vi "URAPI_ForStart.vi"(0 "Iterations":string, 3 "URAPI Script":T1={"Script"="", "Whiles"=[], "Ifs"=[], "Supress Err"=TRUE, "Errors"=""}) -> (2 "variable":string, 5 "URAPI Script Out":T1={"Script"="", "Whiles"=[], "Ifs"=[], "Supress Err"=TRUE, "Errors"=""})   [LabVIEW 2012]
doc: "Begins the execution of a for loop. The loop will execute the specified number of \"iterations\".\nNote: requires Loop end VI."
uses:
  <userlib>/BotSpeak/VIs/Direct/URAPI_Control.ctl
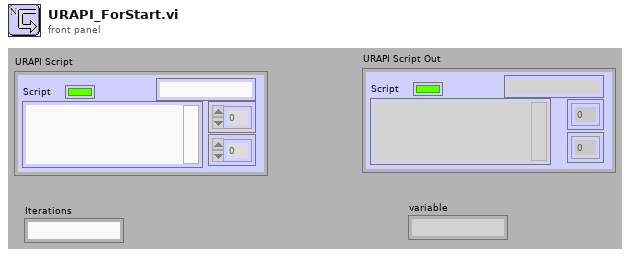
[diagram p1: front panel]
types:
  T1 = typedef "URAPI_Control.ctl" = cluster{"Script":string, "Whiles":u8[], "Ifs":u8[], "Supress Err":bool, "Errors":string}
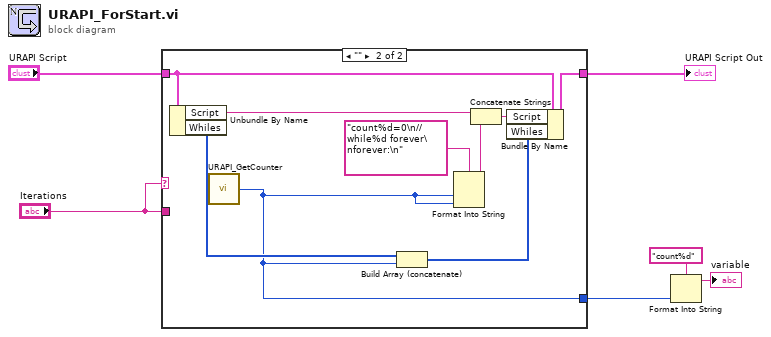
[diagram p0: block diagram]
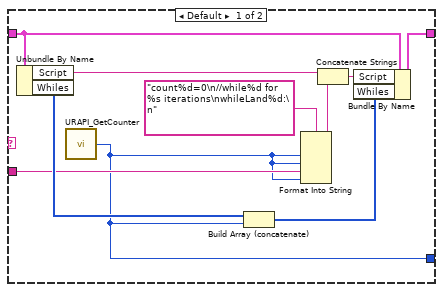
[diagram p2: hidden frame]
diagram:
  n1 = case shown="\"\"" "Iterations" {
    tunnel: "URAPI Script" -> [w16 w25]
    tunnel: [w14 w23] -> w6
    tunnel: "Iterations" -> [w8 _]
    tunnel: [w7 w17] -> w4
    frame Default {
      n2 = Unbundle By Name(w16) -> ("Script"=w11:string, "Whiles"=w10:u8[])
      n3 = call <userlib>:"URAPI_GetCounter.vi"() -> ("Numeric"=w7:u16)  [unwired: 1 in]
      n4 = Build Array (concatenate)(w10, w7) -> (w9:u16[])
      n5 = Format Into String(format string="count%d=0\n//while%d for %s iterations\nwhileLand%d:\n" ("string"), w7, w7, w8, w7) -> (resulting string=w12:string)  [unwired: 2 in, 1 out]
      n6 = Concatenate Strings(w11, w12) -> (w15:string)
      n7 = Bundle By Name(cluster=w16, "Script"=w15, "Whiles"=w9) -> (w14:T1)
    }
    frame "" {
      n8 = Unbundle By Name(w25) -> ("Script"=w20:string, "Whiles"=w19:u8[])
      n9 = call <userlib>:"URAPI_GetCounter.vi"() -> ("Numeric"=w17:u16)  [unwired: 1 in]
      n10 = Build Array (concatenate)(w19, w17) -> (w18:u16[])
      n11 = Format Into String(format string="count%d=0\n//while%d forever\nforever:\n" ("string"), w17, w17) -> (resulting string=w21:string)  [unwired: 2 in, 1 out]
      n12 = Concatenate Strings(w20, w21) -> (w24:string)
      n13 = Bundle By Name(cluster=w25, "Script"=w24, "Whiles"=w18) -> (w23:T1)
    }
  }
  "URAPI Script Out" <- w6
  n14 = Format Into String(format string="count%d", w4) -> (resulting string=→"variable":string)  [unwired: 2 in, 1 out]
